vi "SDT_ReadSetUpBlock.vi"(8 "error in":errorcluster, 10 "bhfile_header":T7 {"chksum" format="x%x"; "header_valid" format="x%x"}, 11 "SDTFileRefnum":refnum<file>) -> (0 "error out":errorcluster, 1 "SetUp":string, 2 "FileInfo":string, 3 "SDTFileRefnum":refnum<file>, 4 "SetUpLength":i32, 5 "MagicNum":u16 format="%x", 6 "BinarySetup_length":u16, 7 "BinarySetupClusters":T6)   [LabVIEW 2023]
doc: "This VI is a SubVI to SDT_ReadFile.vi . It reads the ASCII- and first part of the binary-SetUp block in a SDT-file from disc.\nSee also a different approach at \\Public\\Data\\SPC Files\\SPCGetTimeScaleFromSETfile.vi.\nFor a description of the *.sdt file format see: SPC_data_file_structure.h\n\ninfo@becker-hickl.com"
uses:
  SPC_Wrappers/SPC_Controls/WFParam.ctl
  SPC_Wrappers/SPC_Controls/SPCBinHdrExt.ctl
  SPC_Wrappers/SPC_Controls/SPCBinHdr.ctl
  SPC_Wrappers/SPC_Controls/bhfile_header.ctl
  SPC_Wrappers/SPC_Controls/BHBinHdr.ctl
  SPC_Wrappers/SPC_Controls/SysParExt.ctl
panel:
  out "SysParExt":T4
  out "BHBinHdr":T1
  out "SPCBinHdr":T2
  out "SPCBinHdrExt":T3
  out "WFParam":T5
  out "chksumTopUp":u16 format="%x"
  out "BinarySetUp":string
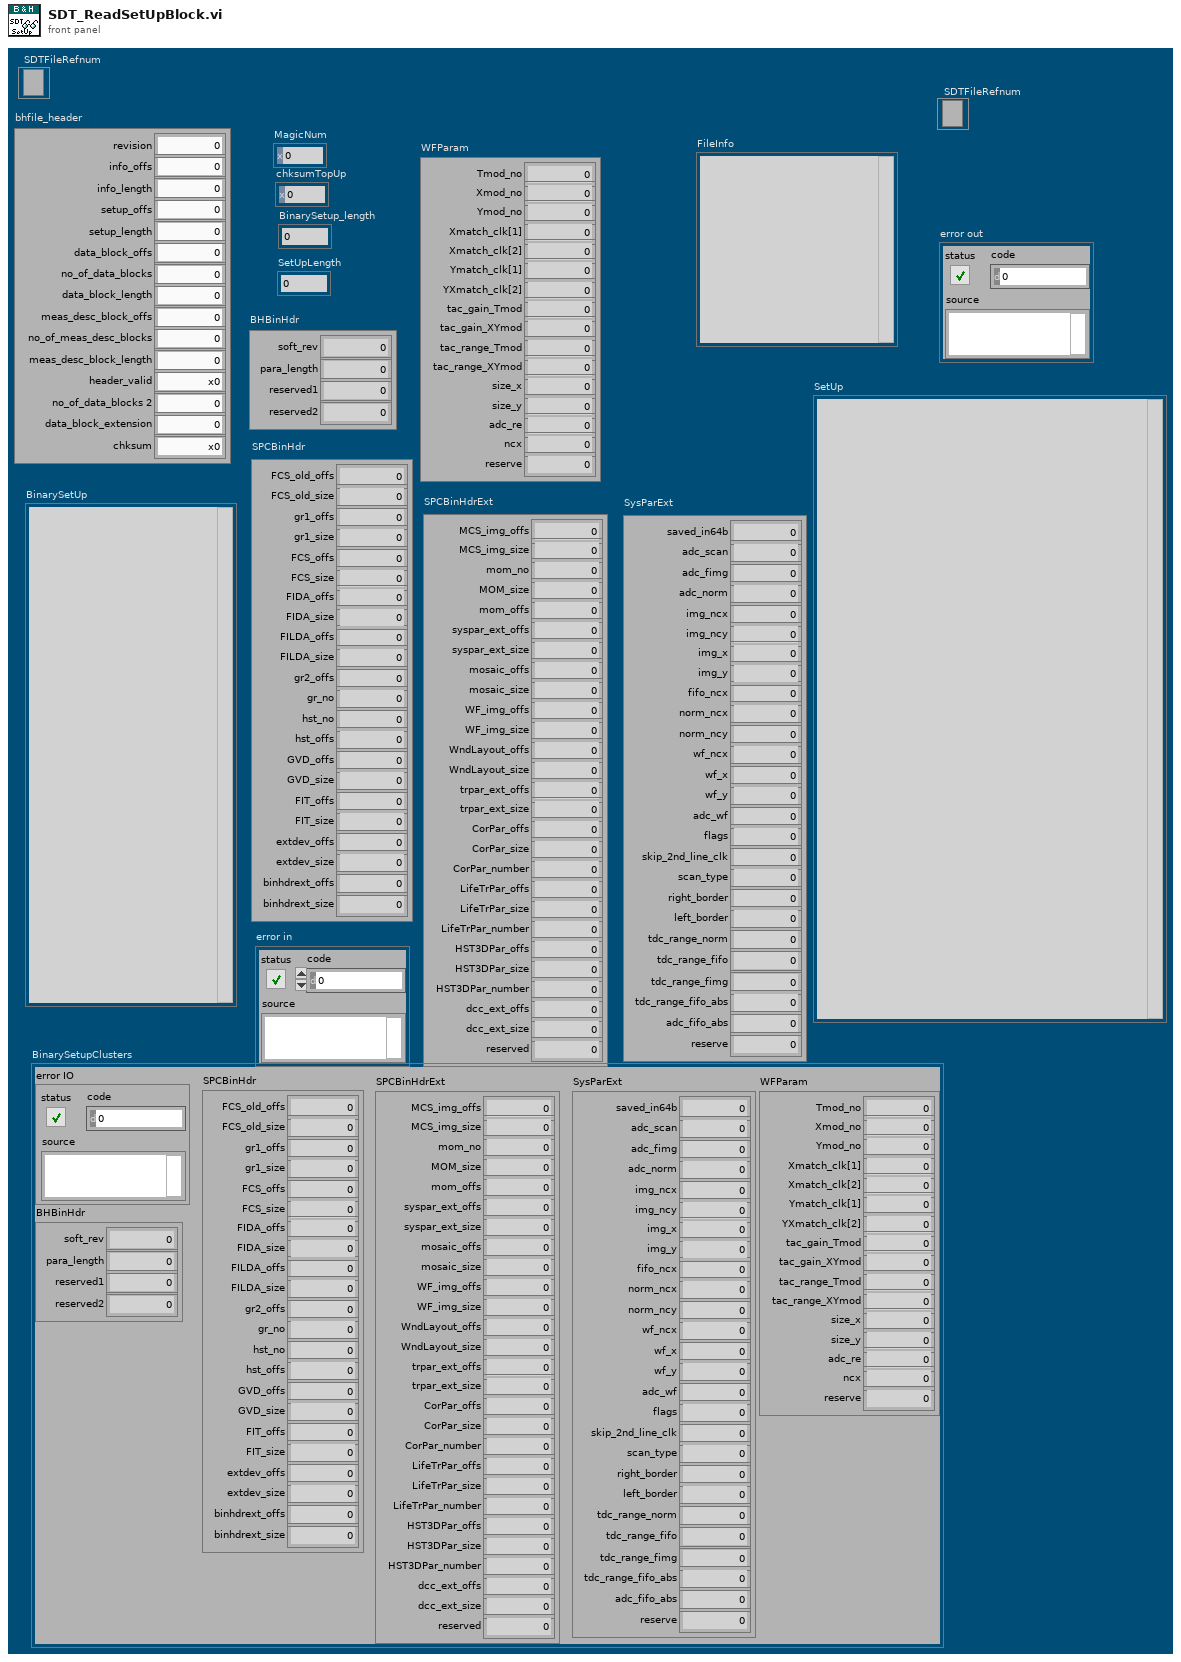
[diagram p1: front panel]
types:
  T1 = typedef "BHBinHdr.ctl" = cluster{"soft_rev":u32, "para_length":u32, "reserved1":u32, "reserved2":u16}
  T2 = typedef "SPCBinHdr.ctl" = cluster{"FCS_old_offs":u32, "FCS_old_size":u32, "gr1_offs":u32, "gr1_size":u32, "FCS_offs":u32, "FCS_size":u32, "FIDA_offs":u32, "FIDA_size":u32, "FILDA_offs":u32, "FILDA_size":u32, "gr2_offs":u32, "gr_no":u16, "hst_no":u16, "hst_offs":u32, "GVD_offs":u32, "GVD_size":u16, "FIT_offs":u16, "FIT_size":u16, "extdev_offs":u16, "extdev_size":u16, "binhdrext_offs":u32, "binhdrext_size":u16}
  T3 = typedef "SPCBinHdrExt.ctl" = cluster{"MCS_img_offs":u32, "MCS_img_size":u32, "mom_no":u16, "MOM_size":u16, "mom_offs":u32, "syspar_ext_offs":u32, "syspar_ext_size":u32, "mosaic_offs":u32, "mosaic_size":u32, "WF_img_offs":u32, "WF_img_size":u16, "WndLayout_offs":u32, "WndLayout_size":u16, "trpar_ext_offs":u32, "trpar_ext_size":u16, "CorPar_offs":u32, "CorPar_size":u16, "CorPar_number":u16, "LifeTrPar_offs":u32, "LifeTrPar_size":u16, "LifeTrPar_number":u16, "HST3DPar_offs":u32, "HST3DPar_size":u16, "HST3DPar_number":u16, "dcc_ext_offs":u32, "dcc_ext_size":u16, "reserved":u16}
  T4 = typedef "SysParExt.ctl" = cluster{"saved_in64b":i16, "adc_scan":i32, "adc_fimg":i32, "adc_norm":i32, "img_ncx":i16, "img_ncy":i16, "img_x":i16, "img_y":i16, "fifo_ncx":i16, "norm_ncx":i16, "norm_ncy":i16, "wf_ncx":i16, "wf_x":i16, "wf_y":i16, "adc_wf":u32, "flags":i16, "skip_2nd_line_clk":i16, "scan_type":i16, "right_border":u32, "left_border":u32, "tdc_range_norm":sgl, "tdc_range_fifo":sgl, "tdc_range_fimg":sgl, "tdc_range_fifo_abs":sgl, "adc_fifo_abs":i32, "reserve":u16}
  T5 = typedef "WFParam.ctl" = cluster{"Tmod_no":i16, "Xmod_no":i16, "Ymod_no":i16, "Xmatch_clk[1]":i16, "Xmatch_clk[2]":i16, "Ymatch_clk[1]":i16, "YXmatch_clk[2]":i16, "tac_gain_Tmod":i16, "tac_gain_XYmod":i16, "tac_range_Tmod":sgl, "tac_range_XYmod":sgl, "size_x":i16, "size_y":i16, "adc_re":i16, "ncx":i16, "reserve":i16}
  T6 = cluster{"error IO":errorcluster, "BHBinHdr":T1, "SPCBinHdr":T2, "SPCBinHdrExt":T3, "SysParExt":T4, "WFParam":T5}
  T7 = typedef "bhfile_header.ctl" = cluster{"revision":i16, "info_offs":i32, "info_length":i16, "setup_offs":i32, "setup_length":u16, "data_block_offs":i32, "no_of_data_blocks":i16, "data_block_length":u32, "meas_desc_block_offs":i32, "no_of_meas_desc_blocks":i16, "meas_desc_block_length":i16, "header_valid":u16, "no_of_data_blocks 2":u32, "data_block_extension":u16, "chksum":u16}
  T8 = enum16{"big-endian, network order", "native, host order", "little-endian"}
  T9 = cluster{bool, "sum":i32, "regular expression":string}
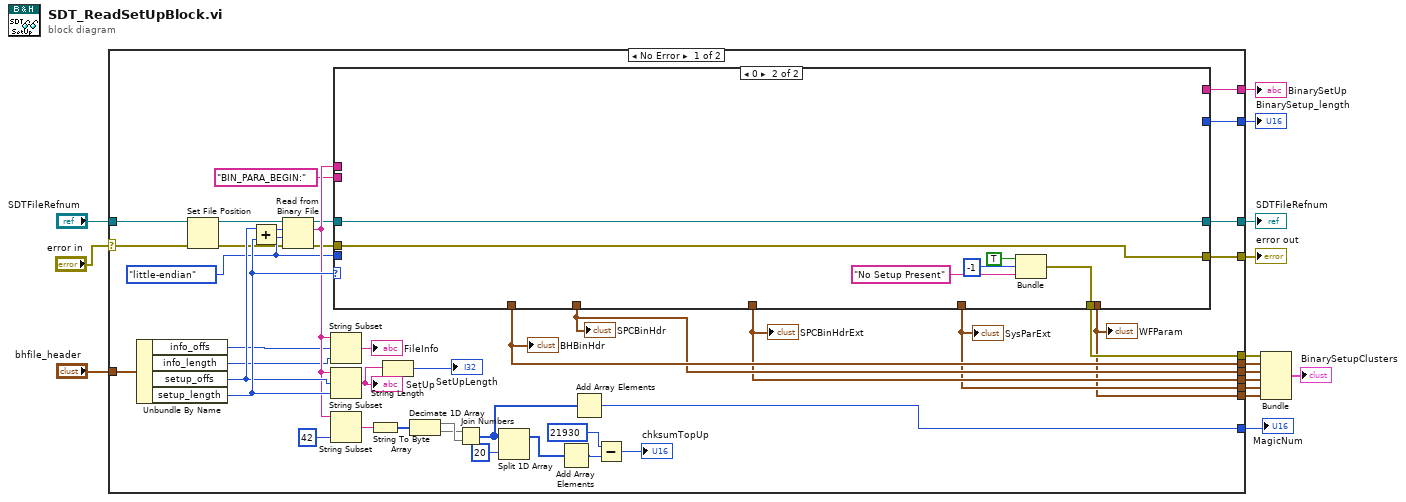
[diagram p0: block diagram]
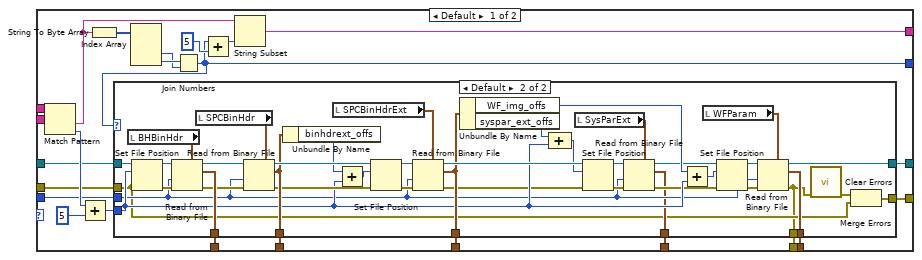
[diagram p2: hidden frame]
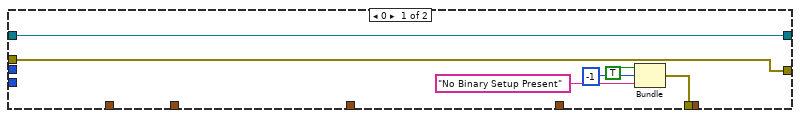
[diagram p3: hidden frame]
diagram:
  n1 = case shown="No Error" "error in" {
    selector: "error in" -> [w26 w132]
    tunnel: [w51 _] -> w15
    tunnel: [w50 _] -> w14
    tunnel: "bhfile_header" -> [w30 _]
    tunnel: "SDTFileRefnum" -> [w29 w133]
    tunnel: [w28 w133] -> w11
    tunnel: [w23 w132] -> w9
    tunnel: [w22 _] -> w8
    tunnel: [w21 w132] -> w7
    tunnel: [w20 _] -> w6
    tunnel: [w19 _] -> w5
    tunnel: [w18 _] -> w4
    tunnel: [w17 _] -> w3
    tunnel: [w16 _] -> w2
    frame No Error {
      w27 = T8."little-endian" ("byte order (0:big-endian, network order)")
      n2 = Unbundle By Name(w30) -> ("info_offs"=w33:i32, "info_length"=w34:i16, "setup_offs"=w52:i32, "setup_length"=w53:u16)
      n3 = Set File Position(refnum=w29, error in=w26) -> (refnum out=w35:refnum<file>, error out=w25:errorcluster)  [unwired: 2 in]
      n4 = Add(x=w52, y=w53) -> (x+y=w36:i32)
      n5 = Read from Binary File(8:w25, 9:w27, 10:w36, 11:w35) -> (0:w24:errorcluster, 2:w38:string, 3:w37:refnum<file>)  [unwired: 2 in, 1 out]
      n6 = String Subset(string=w38, offset (0)=w33, length (rest)=w34) -> (substring=→"FileInfo":string)
      n7 = String Subset(string=w38, offset (0)=w52, length (rest)=w53) -> (substring=w54:string)
      "SetUp" <- w54
      n8 = String Subset(string=w38, length (rest)=42 ("length (rest)")) -> (substring=w40:string)  [unwired: 1 in]
      n9 = case shown="0" w53 {
        tunnel: "BIN_PARA_BEGIN:" ("regular expression") -> [w79 _]
        tunnel: [w69 w131] -> w28
        tunnel: w37 -> [w68 w131]
        tunnel: w27 -> [w62 _]
        tunnel: w38 -> [w67 _]
        tunnel: [w66 _] -> w16
        tunnel: [w65 _] -> w18
        tunnel: [w64 _] -> w19
        tunnel: [w63 _] -> w20
        tunnel: [w58 _] -> w50
        tunnel: [w61 _] -> w51
        tunnel: w24 -> [w60 w130]
        tunnel: [w59 w130] -> w23
        tunnel: [w57 _] -> w17
        tunnel: [w56 w126] -> w21
        frame Default {
          n10 = Match Pattern(string=w67, regular expression=w79) -> (after substring=w75:string, offset past match=w72:i32)  [unwired: 1 in, 2 out]
          n11 = Add(x=w72, y=5) -> (x+y=w70:i32)
          n12 = String To Byte Array(string=w75) -> (unsigned byte array=w78:u8[])
          n13 = Index Array(array=w78) -> (element #2=w76:u8, element #3=w77:u8)  [unwired: 3 in, 1 out]
          n14 = Join Numbers(hi=w77, lo=w76) -> ((hi.lo)=w58:u16)
          n15 = case shown="Default" w58 {
            tunnel: w70 -> [_ w96]
            tunnel: [w84 w116] -> w69
            tunnel: w68 -> [w84 w115]
            tunnel: [_ w114] -> w66
            tunnel: [_ w101] -> w65
            tunnel: [_ w113] -> w64
            tunnel: [_ w112] -> w63
            tunnel: w62 -> [_ w92]
            tunnel: w60 -> [w85 w87]
            tunnel: [w85 w88] -> w59
            tunnel: [_ w90] -> w57
            tunnel: [w80 w86] -> w56
            frame 0 {
              n16 = Bundle(TRUE, "sum"=-1, "regular expression"="No Binary Setup Present") -> (w80:T9)  [unwired: 1 in]
            }
            frame Default {
              n17 = local read "BHBinHdr"() -> (w111:T1)
              n18 = Set File Position(offset (in bytes) (0)=w96, refnum=w115, error in=w87) -> (refnum out=w125:refnum<file>, error out=w107:errorcluster)  [unwired: 1 in]
              n19 = Read from Binary File(5:w111, 8:w107, 9:w92, 11:w125) -> (0:w106:errorcluster, 2:w112:T1, 3:w124:refnum<file>)  [unwired: 2 in, 1 out]
              n20 = local read "SPCBinHdr"() -> (w110:T2)
              n21 = Read from Binary File(5:w110, 8:w106, 9:w92, 11:w124) -> (0:w105:errorcluster, 2:w113:T2, 3:w122:refnum<file>)  [unwired: 2 in, 1 out]
              n22 = Unbundle By Name(w113) -> ("binhdrext_offs"=w119:u32)
              n23 = local read "SPCBinHdrExt"() -> (w109:T3)
              n24 = Add(x=w119, y=w96) -> (x+y=w118:u32)
              n25 = Set File Position(offset (in bytes) (0)=w118, refnum=w122, error in=w105) -> (refnum out=w123:refnum<file>, error out=w104:errorcluster)  [unwired: 1 in]
              n26 = Read from Binary File(5:w109, 8:w104, 9:w92, 11:w123) -> (0:w95:errorcluster, 2:w101:T3, 3:w102:refnum<file>)  [unwired: 2 in, 1 out]
              n27 = Unbundle By Name(w101) -> ("WF_img_offs"=w120:u32, "syspar_ext_offs"=w97:u32)
              n28 = Compound Arithmetic op=ADD(w97, w96) -> (w100:u32)
              n29 = local read "SysParExt"() -> (w91:T4)
              n30 = Set File Position(offset (in bytes) (0)=w100, refnum=w102, error in=w95) -> (refnum out=w99:refnum<file>, error out=w98:errorcluster)  [unwired: 1 in]
              n31 = Read from Binary File(5:w91, 8:w98, 9:w92, 11:w99) -> (0:w94:errorcluster, 2:w90:T4, 3:w93:refnum<file>)  [unwired: 2 in, 1 out]
              n32 = Add(x=w120, y=w96) -> (x+y=w117:u32)
              n33 = local read "WFParam"() -> (w108:T5)
              n34 = Set File Position(offset (in bytes) (0)=w117, refnum=w93, error in=w94) -> (refnum out=w121:refnum<file>, error out=w103:errorcluster)  [unwired: 1 in]
              n35 = Read from Binary File(5:w108, 8:w103, 9:w92, 11:w121) -> (0:w86:errorcluster, 2:w114:T5, 3:w116:refnum<file>)  [unwired: 2 in, 1 out]
              n36 = call <vilib>:"Clear Errors.vi"("error in (no error)"=w86) -> ("error out"=w89:errorcluster)  [unwired: 5 in, 1 out]
              n37 = Merge Errors(w89, w87) -> (w88:errorcluster)
            }
          }
          n38 = Add(x=w58, y=u16 5) -> (x+y=w74:u16)
          n39 = String Subset(string=w75, length (rest)=w74) -> (substring=w61:string)  [unwired: 1 in]
        }
        frame 0 {
          n40 = Bundle(TRUE, "sum"=-1, "regular expression"="No Setup Present") -> (w126:T9)  [unwired: 1 in]
        }
      }
      "SPCBinHdr" <- w19
      "SPCBinHdrExt" <- w18
      "WFParam" <- w16
      "BHBinHdr" <- w20
      "SysParExt" <- w17
      n41 = String To Byte Array(string=w40) -> (unsigned byte array=w41:u8[])
      n42 = String Length(string=w54) -> (length=→"SetUpLength":i32)
      n43 = Decimate 1D Array(w41) -> (w43:u8[], w42:u8[])
      n44 = Join Numbers(hi=w42, lo=w43) -> ((hi.lo)=w45:u16[])
      n45 = Split 1D Array(array=w45, index=20) -> (first subarray=w46:u16[])  [unwired: 1 out]
      n46 = Add Array Elements(numeric array=w46) -> (sum=w47:u16)
      n47 = Add Array Elements(numeric array=w45) -> (sum=w22:u16)
      n48 = Subtract(x=u16 21930 ("y"), y=w47) -> (x-y=→"chksumTopUp":u16)
    }
    frame Error {
    }
  }
  "BinarySetup_length" <- w14
  "BinarySetUp" <- w15
  "SDTFileRefnum" <- w11
  "error out" <- w9
  "MagicNum" <- w8
  n49 = Bundle("error IO"=w7, "BHBinHdr"=w6, "SPCBinHdr"=w5, "SPCBinHdrExt"=w4, "SysParExt"=w3, "WFParam"=w2) -> (→"BinarySetupClusters":T6)  [unwired: 1 in]
